vi "Add Musics To List.vi"(0 "reference in":refnum<class "Client.lvclass">, 5 "Music List":path[](array[path]), 11 "Error In":errorcluster) -> (4 "reference out":refnum<class "Client.lvclass">, 15 "Error Out":errorcluster)   [LabVIEW 2024, in "Client.lvclass"]
uses:
  Client.lvclass
  Client.lvclass/Client.ctl
  Receiver/MediaPlayer_class/MediaPlayer.lvclass
panel:
  # "Connector Pane"
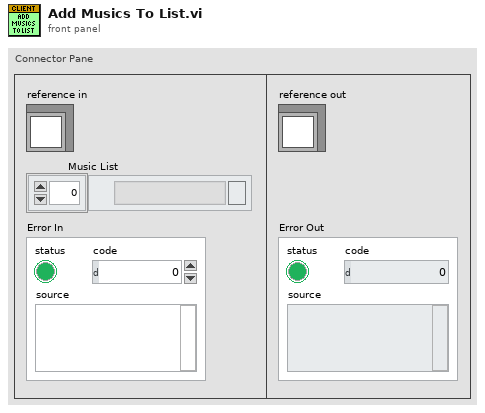
[diagram p1: front panel]
types:
  T1 = typedef "Client.lvclass/ObjectAttributes.ctl" = cluster{"RemoteControlRef":refnum<class "RemoteControl.lvclass">, "MediaPlayerRef":refnum<class "MediaPlayer.lvclass">, "Commands":cluster{"Play Music Command":refnum<class "IPlayerCommand.lvclass">, "Pause Music Command":refnum<class "IPlayerCommand.lvclass">, "Stop Music Command":refnum<class "IPlayerCommand.lvclass">, "Skip Music Command":refnum<class "IPlayerCommand.lvclass">, "Get Current Info Command":refnum<class "IPlayerCommand.lvclass">, "Rewind Music Command":refnum<class "IPlayerCommand.lvclass">}}
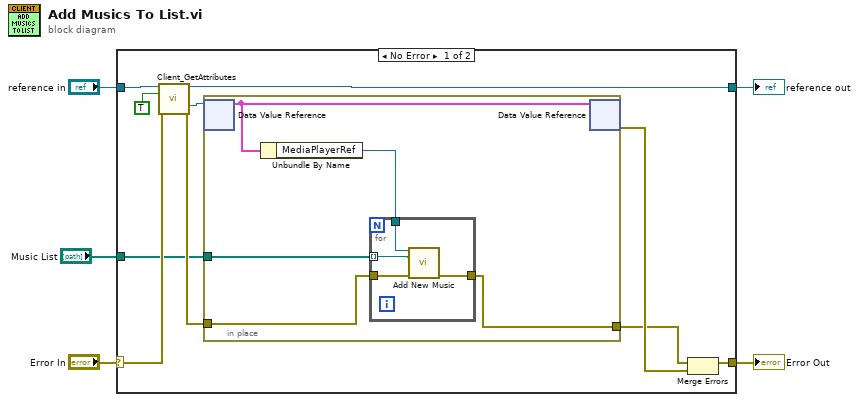
[diagram p0: block diagram]
diagram:
  n1 = case shown="No Error" "Error In" {
    selector: "Error In" -> [w14 w26]
    tunnel: [w11 w26] -> w4
    tunnel: [w12 w25] -> w2
    tunnel: "reference in" -> [w15 w25]
    tunnel: "Music List" -> [w6 _]
    frame No Error {
      n2 = call "Client_GetAttributes.vi"("reference in"=w15, "OnlyGetDvrReference(False)"=TRUE, "Error In"=w14) -> ("reference out"=w12:refnum<class "Client.lvclass">, "DataRef"=w10:refnum<data-value>, "Error Out"=w8:errorcluster)  [unwired: 9 in, 1 out]
      n3 = in-place {
        in-place-border: w8 -> [w18]
        in-place-border: [w17] -> w7
        in-place-border: w6 -> [w16]
        n4 = in-place-dvr #1(w10) -> (w20:T1)  [unwired: 1 out]
        n5 = Unbundle By Name(w20) -> ("MediaPlayerRef"=w19:refnum<class "MediaPlayer.lvclass">)
        n6 = for {
          tunnel: w19 -> [w24]
          tunnel: w18 -> [w23]
          tunnel: [w22] -> w17
          tunnel: w16 -> [w21] mode=indexing
          n7 = call-dynamic "Add New Music.vi"("reference in"=w24, "Music Path"=w21, "Error In"=w23) -> ("Error Out"=w22:errorcluster)  [unwired: 11 in, 1 out]
        }
        n8 = in-place-dvr #1(w20) -> (w13:errorcluster)  [unwired: 1 out]
      }
      n9 = Merge Errors(w7, w13) -> (w11:errorcluster)
    }
    frame Error {
    }
  }
  "Error Out" <- w4
  "reference out" <- w2
